vi "SCTL Sector Accumulation Pipelined.vi"() -> (3 "New Data?":bool)   [LabVIEW 2013]
uses:
  <vilib>/rvi/FIFO/Fifo_Resource/nirvififoEmulationReadFpgaImpl.vi
  <vilib>/rvi/DataTransferAndStorage/Container/Common/niFpgaContainerGetUniqueNameForEmu.vi
  <vilib>/rvi/Memory/Memory_Emulation/nirvimemoryFastEmulationFpgaImpl.vi
  <instcachedir>/0/nirvimemoryFastEmulationFpgaImpl_5FBAB50466BC4C939F684F8805638BFC.lvgen/nirvimemoryFastEmulationFpgaImpl_5FBAB50466BC4C939F684F8805638BFC_011.vi
  <vilib>/rvi/Memory/Memory_Emulation/nirvimemoryFastEmulation.vi
  <vilib>/rvi/Memory/Memory_Emulation/nirvimemoryEmulation.vi
  <vilib>/rvi/DataTransferAndStorage/Container/XNode/niFpgaContainer.xnode
  <vilib>/rvi/FIFO/Fifo_Resource/nirvififoEmulationRead.vi
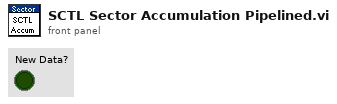
[diagram p1: front panel]
types:
  T1 = cluster{"Accumulated Intensity":u32, "Count":u16}
  T2 = cluster{"Accumulated Intensity":u32, "Count":u16}[]
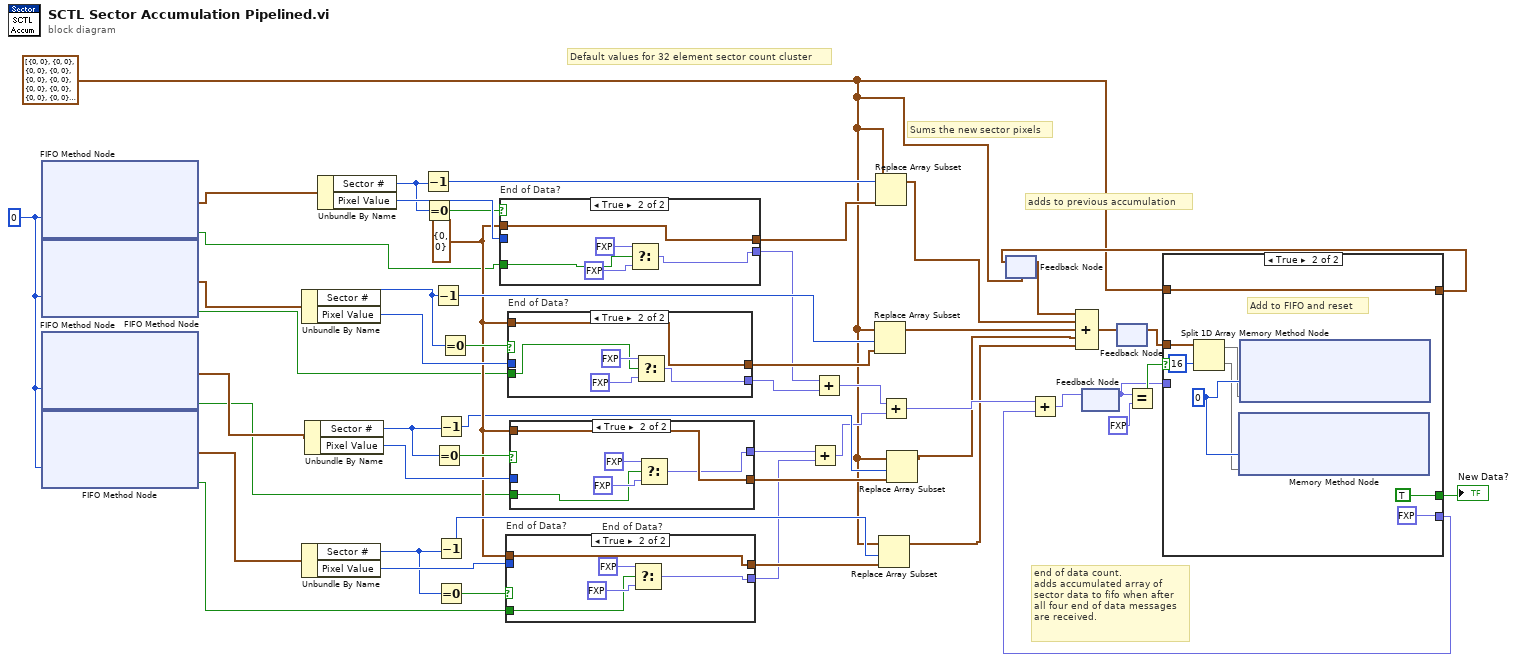
[diagram p0: block diagram]
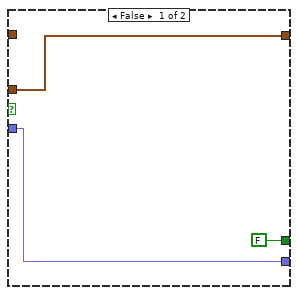
[diagram p2: hidden frame]
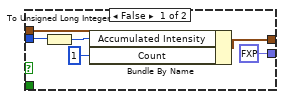
[diagram p3: hidden frame]
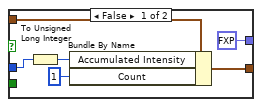
[diagram p4: hidden frame]
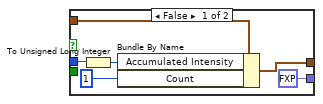
[diagram p5: hidden frame]
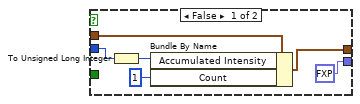
[diagram p6: hidden frame]
diagram:
  w28 = T1 {"Accumulated Intensity"=0, "Count"=0} ("Accumulated Sector Cluster")
  w3 = T2 [{"Accumulated Intensity"=0, "Count"=0}, {"Accumulated Intensity"=0, "Count"=0}, {"Accumulated Intensity"=0, "Count"=0}, {"Accumulated Intensity"=0, "Count"=0}, {"Accumulated Intensity"=0, "Count"=0}, {"Accumulated Intensity"=0, "Count"=0}, {"Accumulated Intensity"=0, "Count"=0}, {"Accumulated Intensity"=0, "Count"=0}, {"Accumulated Intensity"=0, "Count"=0}, {"Accumulated Intensity"=0, "Count"=0}, {"Accumulated Intensity"=0, "Count"=0}, {"Accumulated Intensity"=0, "Count"=0}, {"Accumulated Intensity"=0, "Count"=0}, {"Accumulated Intensity"=0, "Count"=0}, {"Accumulated Intensity"=0, "Count"=0}, {"Accumulated Intensity"=0, "Count"=0}, {"Accumulated Intensity"=0, "Count"=0}, {"Accumulated Intensity"=0, "Count"=0}, {"Accumulated Intensity"=0, "Count"=0}, {"Accumulated Intensity"=0, "Count"=0}, {"Accumulated Intensity"=0, "Count"=0}, {"Accumulated Intensity"=0, "Count"=0}, {"Accumulated Intensity"=0, "Count"=0}, {"Accumulated Intensity"=0, "Count"=0}, {"Accumulated Intensity"=0, "Count"=0}, {"Accumulated Intensity"=0, "Count"=0}, {"Accumulated Intensity"=0, "Count"=0}, {"Accumulated Intensity"=0, "Count"=0}, {"Accumulated Intensity"=0, "Count"=0}, {"Accumulated Intensity"=0, "Count"=0}, {"Accumulated Intensity"=0, "Count"=0}, {"Accumulated Intensity"=0, "Count"=0}] ("Data")
  w52 = 0 ("Timeout")
  # "end of data count.\nadds accumulated array of\nsector data to fifo when after\nall four end of data messages\nare received."
  # "adds to previous accumulation"
  # "Sums the new sector pixels"
  # "Default values for 32 element sector count cluster"
  n1 = xnode ("FIFO Method Node")("Timeout"=w52) -> ("Element"=w24:cluster{"Sector #":u8, "Pixel Value":u8}, "Timed Out?"=w20:bool)  [unwired: 1 in, 1 out]
  n2 = xnode ("FIFO Method Node")("Timeout"=w52) -> ("Element"=w23:cluster{"Sector #":u8, "Pixel Value":u8}, "Timed Out?"=w19:bool)  [unwired: 1 in, 1 out]
  n3 = xnode ("FIFO Method Node")("Timeout"=w52) -> ("Element"=w22:cluster{"Sector #":u8, "Pixel Value":u8}, "Timed Out?"=w18:bool)  [unwired: 1 in, 1 out]
  n4 = xnode ("FIFO Method Node")("Timeout"=w52) -> ("Element"=w21:cluster{"Sector #":u8, "Pixel Value":u8}, "Timed Out?"=w17:bool)  [unwired: 1 in, 1 out]
  n5 = Unbundle By Name(w23) -> ("Sector #"=w38:u8, "Pixel Value"=w48:u8)
  n6 = Unbundle By Name(w21) -> ("Sector #"=w34:u8, "Pixel Value"=w42:u8)
  n7 = Unbundle By Name(w22) -> ("Sector #"=w36:u8, "Pixel Value"=w45:u8)
  n8 = Unbundle By Name(w24) -> ("Sector #"=w40:u8, "Pixel Value"=w50:u8)
  n9 = Decrement(x=w40) -> (x-1=w51:u8)
  n10 = Equal To 0?(x=w40) -> (x = 0?=w39:bool)
  n11 = Decrement(x=w38) -> (x-1=w47:u8)
  n12 = Equal To 0?(x=w36) -> (x = 0?=w35:bool)
  n13 = Decrement(x=w36) -> (x-1=w26:u8)
  n14 = Decrement(x=w34) -> (x-1=w44:u8)
  n15 = Equal To 0?(x=w34) -> (x = 0?=w33:bool)
  n16 = Equal To 0?(x=w38) -> (x = 0?=w37:bool)
  n17 = case "End of Data?" shown="True" w39 {
    tunnel: w50 -> [w54 _]
    tunnel: [w58 w63] -> w49
    tunnel: w28 -> [w57 w63]
    tunnel: [fxp<+,1,1> 0.0 w59] -> w16
    tunnel: w20 -> [_ w62]
    frame False {
      n18 = To Unsigned Long Integer(number=w54) -> (unsigned 32bit integer=w53:u32)
      n19 = Bundle By Name(cluster=w57, "Accumulated Intensity"=w53, "Count"=u16 1) -> (w58:T1)
    }
    frame True {
      n20 = Select(t=fxp<+,1,1> 0.0, s=w62, f=fxp<+,1,1> 1.0) -> (s? t:f=w59:fxp<+,1,1>)
    }
  }
  n21 = case "End of Data?" shown="True" w33 {
    tunnel: [w69 w74] -> w43
    tunnel: w28 -> [w68 w74]
    tunnel: w42 -> [w65 _]
    tunnel: [fxp<+,1,1> 0.0 w70] -> w13
    tunnel: w17 -> [_ w71]
    frame False {
      n22 = To Unsigned Long Integer(number=w65) -> (unsigned 32bit integer=w64:u32)
      n23 = Bundle By Name(cluster=w68, "Accumulated Intensity"=w64, "Count"=u16 1) -> (w69:T1)
    }
    frame True {
      n24 = Select(t=fxp<+,1,1> 0.0, s=w71, f=fxp<+,1,1> 1.0) -> (s? t:f=w70:fxp<+,1,1>)
    }
  }
  n25 = case "End of Data?" shown="True" w37 {
    tunnel: w48 -> [w76 _]
    tunnel: w28 -> [w80 w85]
    tunnel: [w79 w85] -> w41
    tunnel: [fxp<+,1,1> 0.0 w81] -> w15
    tunnel: w19 -> [_ w82]
    frame False {
      n26 = To Unsigned Long Integer(number=w76) -> (unsigned 32bit integer=w75:u32)
      n27 = Bundle By Name(cluster=w80, "Accumulated Intensity"=w75, "Count"=u16 1) -> (w79:T1)
    }
    frame True {
      n28 = Select(t=fxp<+,1,1> 0.0, s=w82, f=fxp<+,1,1> 1.0) -> (s? t:f=w81:fxp<+,1,1>)
    }
  }
  n29 = case "End of Data?" shown="True" w35 {
    tunnel: [w91 w96] -> w46
    tunnel: w45 -> [w87 _]
    tunnel: w28 -> [w90 w96]
    tunnel: [fxp<+,1,1> 0.0 w92] -> w14
    tunnel: w18 -> [_ w93]
    frame False {
      n30 = To Unsigned Long Integer(number=w87) -> (unsigned 32bit integer=w86:u32)
      n31 = Bundle By Name(cluster=w90, "Accumulated Intensity"=w86, "Count"=u16 1) -> (w91:T1)
    }
    frame True {
      n32 = Select(t=fxp<+,1,1> 0.0, s=w93, f=fxp<+,1,1> 1.0) -> (s? t:f=w92:fxp<+,1,1>)
    }
  }
  n33 = Add(x=w14, y=w13) -> (x+y=w11:fxp<+,2,2>)
  n34 = Add(x=w16, y=w15) -> (x+y=w12:fxp<+,2,2>)
  n35 = Replace Array Subset(array=w3, new element=w41, index=w47) -> (w5:T2)
  n36 = Replace Array Subset(array=w3, new element=w49, index=w51) -> (w4:T2)
  n37 = Replace Array Subset(array=w3, new element=w43, index=w44) -> (w7:T2)
  n38 = Add(x=w12, y=w11) -> (x+y=w10:fxp<+,3,3>)
  n39 = Replace Array Subset(array=w3, new element=w46, index=w26) -> (w6:T2)
  n40 = feedback #1(w3) -> (w25:T2)
  n41 = Compound Arithmetic op=ADD(w25, w4, w5, w6, w7) -> (w2:T2)
  n42 = feedback #2() -> (w30:fxp<+,3,3>)  [unwired: 1 in]
  n43 = feedback #3() -> (w1:T2)  [unwired: 1 in]
  n44 = feedback-in #3(w2) -> ()
  n45 = Equal?(x=w30, y=fxp<+,3,3> 4.0) -> (x = y?=w31:bool)
  n46 = case shown="True" w31 {
    tunnel: w1 -> [w99 w104]
    tunnel: [w97 fxp<+,3,3> 0.0] -> w9
    tunnel: w30 -> [w97 _]
    tunnel: [w99 w106] -> w29
    tunnel: w3 -> [_ w106]
    tunnel: [FALSE ("New Data?") TRUE ("New Data?")] -> w27
    frame False {
    }
    frame True {
      w105 = 0 ("Timeout")
      # "Add to FIFO and reset"
      n47 = Split 1D Array(array=w104, index=16) -> (first subarray=w102:T2, second subarray=w101:T2)
      n48 = xnode ("Memory Method Node")("Address"=w105, "Data"=w101) -> ()  [unwired: 1 in, 1 out]
      n49 = xnode ("Memory Method Node")("Address"=w105, "Data"=w102) -> ()  [unwired: 1 in, 1 out]
    }
  }
  "New Data?" <- w27
  n50 = feedback-in #1(w29) -> ()
  n51 = Add(x=w10, y=w9) -> (x+y=w8:fxp<+,3,3>)
  n52 = feedback-in #2(w8) -> ()
